vi "Overview.vi"() -> ()   [LabVIEW 2023, in "SQL Database.lvlib"]
uses:
  SQL Database.lvlib
  <vilib>/addons/database/NI_Database_API.lvlib
  <vilib>/addons/database/_DB Variant To Data/Database Variant To Data.xnode
  <vilib>/addons/database/Connection.llb/DB Tools Open Connec (Path).vi
  <vilib>/addons/database/Connection.llb/Conn Execute.vi
  <vilib>/addons/database/Recordset.llb/Rec Fetch Recordset Data (R).vi
  <vilib>/addons/database/Recordset.llb/Rec Fetch String Data (R).vi
  <vilib>/addons/database/Recordset.llb/Rec Move To Previous Record (R).vi
  <vilib>/addons/database/Command.llb/Cmd Set Parameter Value (CR).vi
  <vilib>/addons/database/Recordset.llb/Rec Move To Next Record (CR).vi
  <vilib>/addons/database/Command.llb/Cmd Get String Parameter Value (C).vi
  <vilib>/addons/database/Recordset.llb/Rec Fetch Next Recordset (R).vi
  <vilib>/addons/database/Command.llb/Cmd Delete.vi
  <vilib>/addons/database/Connection.llb/Conn Get Properties.vi
  <vilib>/addons/database/Auxilliary.llb/DB Tools Format Datetime String (Time Stamp).vi
  <vilib>/addons/database/Connection.llb/Conn Transaction.vi
  <vilib>/addons/database/Recordset.llb/Rec Save Recordset To File (R).vi
  <vilib>/addons/database/Connection.llb/Conn Set Properties.vi
  <vilib>/addons/database/Auxilliary.llb/DB Tools DataTypes.ctl
  <vilib>/addons/database/Auxilliary.llb/DB Tools Column Info.ctl
  <vilib>/addons/database/Auxilliary.llb/DB Tools Cursor Type.ctl
  <vilib>/addons/database/Auxilliary.llb/DB Tools Parameter Dir.ctl
  <vilib>/addons/database/Auxilliary.llb/DB Tools Parameter Info.ctl
  <vilib>/addons/database/Connection.llb/Conn Properties.ctl
panel:
  out "date/time string":string
  in  "time stamp":timestamp
  out "connection properties 2":T1
  in  "connection properties":T1
  in  "value":variant
  in  "parameter index":variant
  in  "parameters":T2[](array[typedef])
  in  "type":string
  in  "column index":variant
  in  "cache size (1)":i32=1 min=1
  in  "cursor type":T5
  in  "SQL query":string
  out "recordset data":variant[][](array[variant])
  out "data 3":variant
  in  "primary key (-1)":i32=-1
  in  "table 4":string
  in  "table 3":string
  out "data 2":variant[][](array[variant])
  in  "columns 2":string[](array[string])
  in  "table 2":string
  in  "condition":string
  in  "data":variant
  in  "columns":string[](array[string])
  in  "table":string
  in  "connection information":path
  in  "column information":T6[](array[typedef])
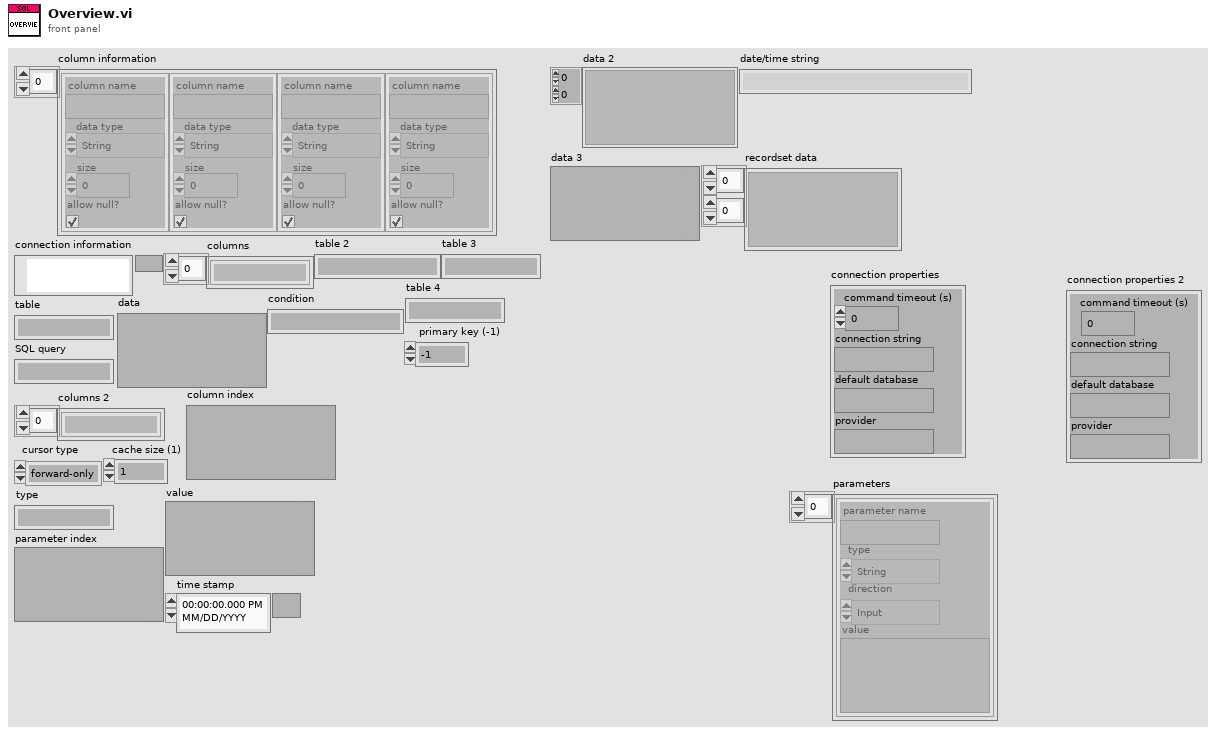
[diagram p1: front panel]
types:
  T1 = typedef "NI_Database_API.lvlib/Conn Properties.ctl" = cluster{"command timeout (s)":i32, "connection string":string, "default database":string, "provider":string}
  T2 = typedef "NI_Database_API.lvlib/DB Tools Parameter Info.ctl" = cluster{"parameter name":string, "type":T3, "direction":T4, "value":variant}
  T3 = typedef "NI_Database_API.lvlib/DB Tools DataTypes.ctl" = enum16{"String", "Long (I32)", "Single (SGL)", "Double (DBL)", "Date/Time", "Binary"}
  T4 = typedef "NI_Database_API.lvlib/DB Tools Parameter Dir.ctl" = enum32{"Input", "Output", "Input/Output", "Return Value"}
  T5 = typedef "NI_Database_API.lvlib/DB Tools Cursor Type.ctl" = enum16{"forward-only", "keyset", "dynamic", "static"}
  T6 = typedef "NI_Database_API.lvlib/DB Tools Column Info.ctl" = cluster{"column name":string, "data type":T3, "size":i32, "allow null?":bool}
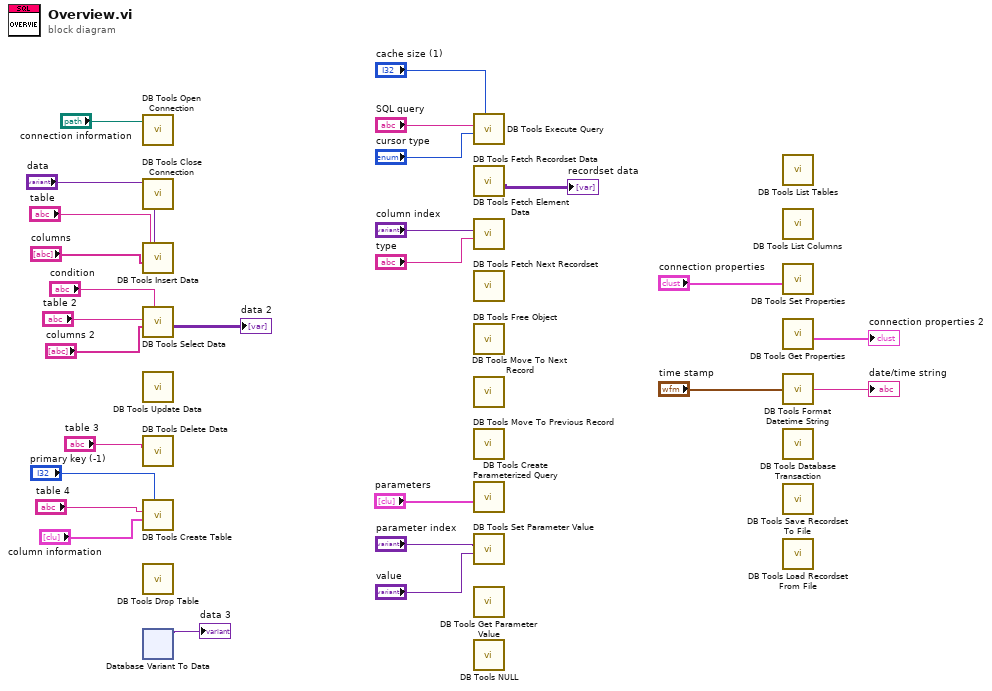
[diagram p0: block diagram]
diagram:
  n1 = call-poly <vilib>:"DB Tools Open Connection.vi"("connection information"="connection information") -> ()  [unwired: 7 in, 2 out]
  n2 = call <vilib>:"DB Tools Close Connection.vi"() -> ()  [unwired: 7 in, 1 out]
  n3 = call <vilib>:"DB Tools Insert Data.vi"("data"="data", "columns"="columns", "table"="table") -> ()  [unwired: 7 in, 2 out]
  n4 = call <vilib>:"DB Tools Select Data.vi"("condition"="condition", "columns"="columns 2", "table"="table 2") -> ("data"=→"data 2":variant[][])  [unwired: 3 in, 2 out]
  n5 = call <vilib>:"DB Tools Update Data.vi"() -> ()  [unwired: 10 in, 2 out]
  n6 = call <vilib>:"DB Tools Delete Data.vi"("table"="table 3") -> ()  [unwired: 9 in, 2 out]
  n7 = call <vilib>:"DB Tools Create Table.vi"("primary key (-1)"="primary key (-1)", "column information"="column information", "table"="table 4") -> ()  [unwired: 5 in, 2 out]
  n8 = call <vilib>:"DB Tools Drop Table.vi"() -> ()  [unwired: 8 in, 2 out]
  n9 = xnode "Database Variant To Data"() -> ("data"=→"data 3":variant)  [unwired: 3 in, 1 out]
  n10 = call-poly <vilib>:"DB Tools Execute Query.vi"("cache size (1)"="cache size (1)", "cursor type"="cursor type", "SQL query"="SQL query") -> ()  [unwired: 5 in, 2 out]
  n11 = call-poly <vilib>:"DB Tools Fetch Recordset Data.vi"() -> ("recordset data"=→"recordset data":variant[][])  [unwired: 5 in, 2 out]
  n12 = call-poly <vilib>:"DB Tools Fetch Element Data.vi"("type"="type", "column index"="column index") -> ()  [unwired: 5 in, 3 out]
  n13 = call-poly <vilib>:"DB Tools Fetch Next Recordset.vi"() -> ()  [unwired: 6 in, 2 out]
  n14 = call-poly <vilib>:"DB Tools Free Object.vi"() -> ()  [unwired: 10 in, 2 out]
  n15 = call-poly <vilib>:"DB Tools Move To Next Record.vi"() -> ()  [unwired: 10 in, 2 out]
  n16 = call-poly <vilib>:"DB Tools Move To Previous Record.vi"() -> ()  [unwired: 10 in, 2 out]
  n17 = call <vilib>:"DB Tools Create Parameterized Query.vi"("parameters"="parameters") -> ()  [unwired: 6 in, 3 out]
  n18 = call-poly <vilib>:"DB Tools Set Parameter Value.vi"("value"="value", "parameter index"="parameter index") -> ()  [unwired: 6 in, 2 out]
  n19 = call-poly <vilib>:"DB Tools Get Parameter Value.vi"() -> ()  [unwired: 7 in, 3 out]
  n20 = call <vilib>:"DB Tools NULL.vi"() -> ()  [unwired: 10 in, 2 out]
  n21 = call <vilib>:"DB Tools List Tables.vi"() -> ()  [unwired: 5 in, 3 out]
  n22 = call <vilib>:"DB Tools List Columns.vi"() -> ()  [unwired: 4 in, 4 out]
  n23 = call-poly <vilib>:"DB Tools Set Properties.vi"("connection properties"="connection properties") -> ()  [unwired: 5 in, 2 out]
  n24 = call-poly <vilib>:"DB Tools Get Properties.vi"() -> ("connection properties"=→"connection properties 2":T1)  [unwired: 5 in, 2 out]
  n25 = call-poly <vilib>:"DB Tools Format Datetime String.vi"("time stamp"="time stamp") -> ("date/time string"=→"date/time string":string)
  n26 = call-poly <vilib>:"DB Tools Database Transaction.vi"() -> ()  [unwired: 6 in, 2 out]
  n27 = call-poly <vilib>:"DB Tools Save Recordset To File.vi"() -> ()  [unwired: 8 in, 2 out]
  n28 = call <vilib>:"DB Tools Load Recordset From File.vi"() -> ()  [unwired: 6 in, 2 out]
